vi "DragOver Accept Inbetween Calc Wrapper.vi"(8 "Displayed Row":i32, 9 "TreeItem Indices (DragStart)":i32[](array[numeric]), 10 "TreeItem Indices (Displayed Items)":i32[](array[numeric]), 11 "TreeItems":T1[](array[typedef])) -> (3 "max indent allowed":i32)   [LabVIEW 2020, in "BetterDragAndDrop.lvlib" / "BetterTreeHandle.lvclass"]
uses:
  Classes/BetterTreeHandle/BetterTreeHandle.lvclass
  Classes/BetterTreeItem/SubVIs/TreeItem.ctl
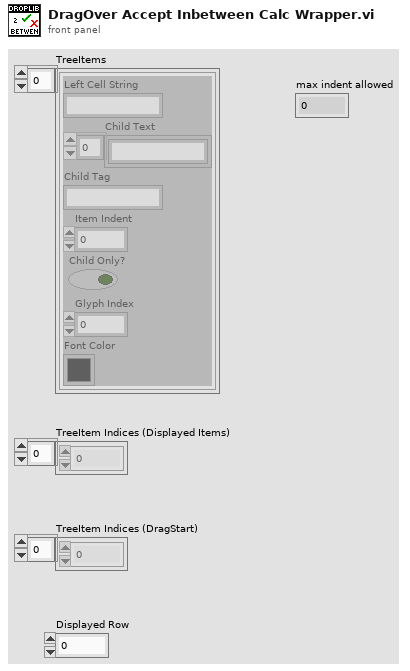
[diagram p1: front panel]
types:
  T1 = typedef "BetterDragAndDrop.lvlib/BetterTreeHandle.lvclass/TreeItem.ctl" = cluster{"Left Cell String":string, "Child Text":string[], "Child Tag":string, "Item Indent":i32, "Child Only?":bool, "Glyph Index":i32, "Font Color":u32}
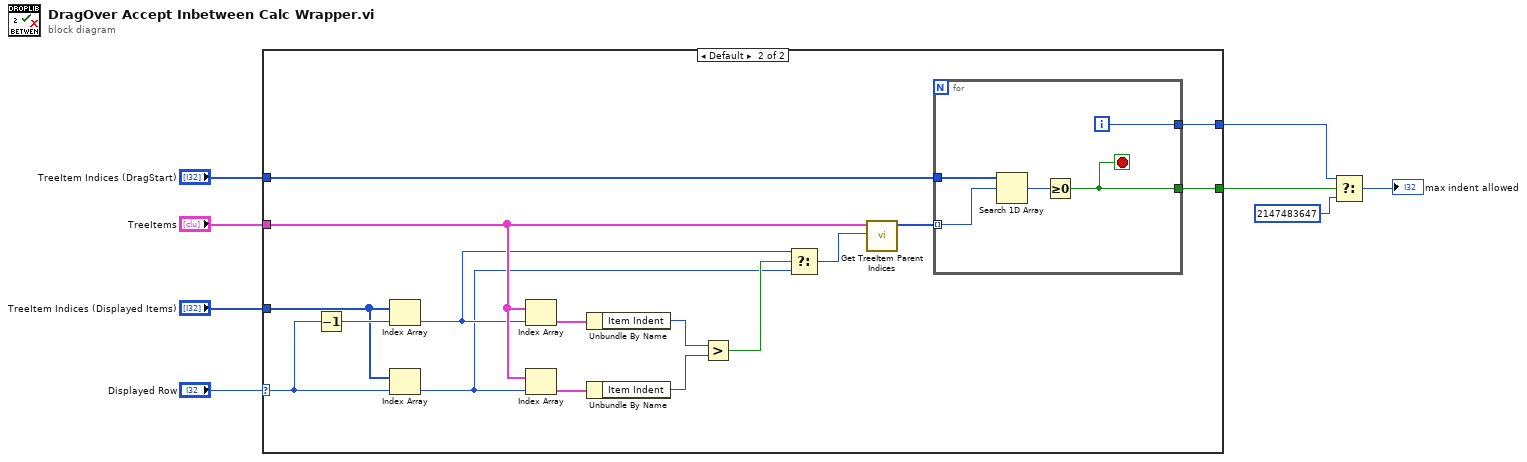
[diagram p0: block diagram]
diagram:
  n1 = case shown="Default" "Displayed Row" {
    selector: "Displayed Row" -> [_ w17]
    tunnel: "TreeItem Indices (Displayed Items)" -> [_ w16]
    tunnel: "TreeItems" -> [_ w15]
    tunnel: "TreeItem Indices (DragStart)" -> [_ w23]
    tunnel: [_ w22] -> w4
    tunnel: [_ w21] -> w2
    frame 0 {
    }
    frame Default {
      n2 = Decrement(x=w17) -> (x-1=w20:i32)
      n3 = Index Array(array=w16, index=w20) -> (element=w11:i32)
      n4 = Index Array(array=w16, index=w17) -> (element=w10:i32)
      n5 = Index Array(array=w15, index=w11) -> (element=w19:T1)
      n6 = Index Array(array=w15, index=w10) -> (element=w18:T1)
      n7 = Unbundle By Name(w19) -> ("Item Indent"=w14:i32)
      n8 = Unbundle By Name(w18) -> ("Item Indent"=w13:i32)
      n9 = Greater?(x=w14, y=w13) -> (0:w12:bool)
      n10 = Select(t=w11, s=w12, f=w10) -> (s? t:f=w9:i32)
      n11 = call "Get TreeItem Parent Indices.vi"("TreeItem Index"=w9, "TreeItems"=w15) -> ("parent indices (incrementing)"=w24:i32[])  [unwired: 8 in, 1 out]
      n12 = for {
        tunnel: w24 -> [w27] mode=indexing
        tunnel: w23 -> [w29]
        tunnel: [w26] -> w22
        tunnel: [w25] -> w21
        i -> [w25]
        stop <- w26 stop-if-true
        n13 = Search 1D Array(1D array=w29, element=w27) -> (index of element=w28:i32)  [unwired: 1 in]
        n14 = Greater Or Equal To 0?(x=w28) -> (x >= 0?=w26:bool)
      }
    }
  }
  n15 = Select(t=w2, s=w4, f=2147483647 ("max indent allowed")) -> (s? t:f=→"max indent allowed":i32)
